vi "VI Tree.vi"   [LabVIEW 2013, in "Ocean Optics 2000 4000.lvlib"]
doc: "This is the instrument driver for the Ocean Optics 2000 4000. The VI Tree displays all the user-callable VIs of the instrument driver in an organized table."
uses:
  <instrlib>/Ocean Optics 2000 4000/Ocean Optics 2000 4000.lvlib
panel:
  # "(c) 2009-2013 National Instruments.  ALL RIGHTS RESERVED."
  # "SEE DIAGRAM\nFOR VI TREE."
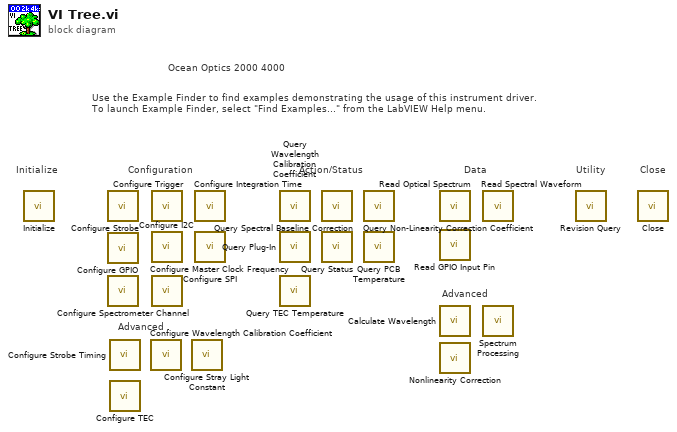
[diagram p0: block diagram]
diagram:
  # "Advanced"
  # "Advanced"
  # "Ocean Optics 2000 4000"
  # "Use the Example Finder to find examples demonstrating the usage of this instrument driver.\nTo launch Example Finder, select \"Find Examples...\" from the LabVIEW Help menu."
  # "Configuration"
  # "Utility"
  # "Data"
  # "Action/Status"
  # "Close"
  # "Initialize"
  n1 = call <instrlib>:"Initialize.vi"() -> ()  [unwired: 10 in, 2 out]
  n2 = call <instrlib>:"Configure Strobe.vi"() -> ()  [unwired: 10 in, 2 out]
  n3 = call <instrlib>:"Configure GPIO.vi"() -> ()  [unwired: 14 in, 2 out]
  n4 = call <instrlib>:"Configure Spectrometer Channel.vi"() -> ()  [unwired: 10 in, 2 out]
  n5 = call <instrlib>:"Configure Strobe Timing.vi"() -> ()  [unwired: 14 in, 2 out]
  n6 = call <instrlib>:"Configure TEC.vi"() -> ()  [unwired: 14 in, 2 out]
  n7 = call <instrlib>:"Configure Wavelength Calibration Coefficient.vi"() -> ()  [unwired: 10 in, 2 out]
  n8 = call <instrlib>:"Configure Trigger.vi"() -> ()  [unwired: 10 in, 2 out]
  n9 = call <instrlib>:"Configure I2C.vi"() -> ()  [unwired: 10 in, 2 out]
  n10 = call <instrlib>:"Configure Master Clock Frequency.vi"() -> ()  [unwired: 10 in, 2 out]
  n11 = call <instrlib>:"Configure Stray Light Constant.vi"() -> ()  [unwired: 10 in, 2 out]
  n12 = call <instrlib>:"Configure Integration Time.vi"() -> ()  [unwired: 10 in, 2 out]
  n13 = call <instrlib>:"Configure SPI.vi"() -> ()  [unwired: 9 in, 3 out]
  n14 = call <instrlib>:"Query Wavelength Calibration Coefficient.vi"() -> ()  [unwired: 6 in, 6 out]
  n15 = call <instrlib>:"Query Plug-In.vi"() -> ()  [unwired: 8 in, 4 out]
  n16 = call <instrlib>:"Query TEC Temperature.vi"() -> ()  [unwired: 9 in, 3 out]
  n17 = call <instrlib>:"Query Spectral Baseline Correction.vi"() -> ()  [unwired: 9 in, 3 out]
  n18 = call <instrlib>:"Query Status.vi"() -> ()  [unwired: 8 in, 8 out]
  n19 = call <instrlib>:"Query Non-Linearity Correction Coefficient.vi"() -> ()  [unwired: 8 in, 4 out]
  n20 = call <instrlib>:"Query PCB Temperature.vi"() -> ()  [unwired: 9 in, 3 out]
  n21 = call <instrlib>:"Read Optical Spectrum.vi"() -> ()  [unwired: 8 in, 4 out]
  n22 = call <instrlib>:"Read GPIO Input Pin.vi"() -> ()  [unwired: 9 in, 3 out]
  n23 = call <instrlib>:"Calculate Wavelength.vi"() -> ()  [unwired: 9 in, 3 out]
  n24 = call <instrlib>:"Nonlinearity Correction.vi"() -> ()  [unwired: 9 in, 3 out]
  n25 = call <instrlib>:"Read Spectral Waveform.vi"() -> ()  [unwired: 9 in, 3 out]
  n26 = call <instrlib>:"Spectrum Processing.vi"() -> ()  [unwired: 13 in, 3 out]
  n27 = call <instrlib>:"Revision Query.vi"() -> ()  [unwired: 7 in, 5 out]
  n28 = call <instrlib>:"Close.vi"() -> ()  [unwired: 11 in, 1 out]
